vi "Hello.vi"(10 "error in (no error)":errorcluster, 11 "WAMP Client in":refnum<class "WAMP Client.lvclass">) -> (0 "Session ID":u32, 1 "<JSON>":string[](array[string]), 2 "error out":errorcluster, 3 "WAMP Client out":refnum<class "WAMP Client.lvclass">)   [LabVIEW 2020, in "WAMP Client.lvclass"]
uses:
  <userlib>/lvwamp/WAMP Client/WAMP Client.lvclass
  <userlib>/lvwamp/WAMP Client/WAMP Client.lvclass/WAMP Client.ctl
  81aa3083-7749-3644-b591-d0aa62dd8321.vi
  <vilib>/JDP Science/JSONtext/JSON text to Variant.vi
  <vilib>/JDP Science/JSONtext/LVClass Serializer/JSONtext LVClass Serializer.lvclass
  <userlib>/lvwamp/Comm Handlers/ICommHandler/ICommHandler.lvclass
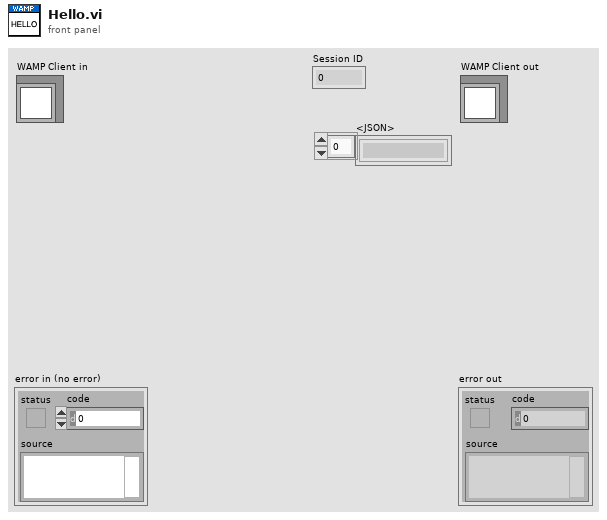
[diagram p1: front panel]
types:
  T1 = typedef "WAMP Client.lvclass/MessageCodes.ctl" = u16
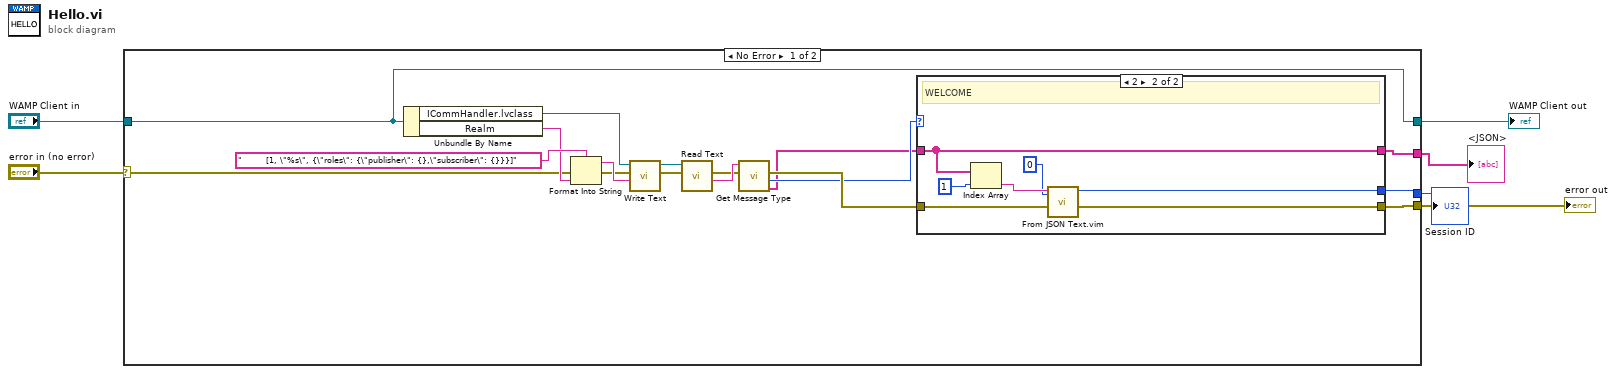
[diagram p0: block diagram]
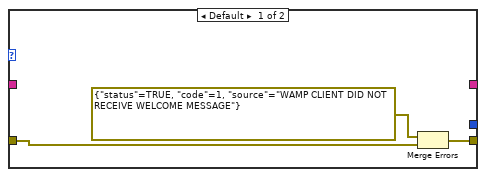
[diagram p2: hidden frame]
diagram:
  n1 = case shown="No Error" "error in (no error)" {
    selector: "error in (no error)" -> [w16 w35]
    tunnel: [w14 w35] -> w5
    tunnel: [w20 w34] -> w3
    tunnel: "WAMP Client in" -> [w20 w34]
    tunnel: [w7 _] -> w2
    tunnel: [w8 _] -> w1
    frame No Error {
      n2 = Unbundle By Name(w20) -> ("ICommHandler.lvclass"=w21:refnum<class "ICommHandler.lvclass">, "Realm"=w18:string)
      n3 = Format Into String(format string="        [1, \"%s\", {\"roles\": {\"publisher\": {},\"subscriber\": {}}}]", error in=w16, w18) -> (resulting string=w17:string, error out=w15:errorcluster)  [unwired: 1 in]
      n4 = call-dynamic "Write Text.vi"("String"=w17, "error in (no error)"=w15, "ICommHandler in"=w21) -> ("error out"=w22:errorcluster, "ICommHandler out"=w23:refnum<class "ICommHandler.lvclass">)  [unwired: 7 in]
      n5 = call-dynamic "Read Text.vi"("error in (no error)"=w22, "ICommHandler in"=w23) -> ("String"=w13:string, "error out"=w12:errorcluster)  [unwired: 5 in, 1 out]
      n6 = call <userlib>:"Get Message Type.vi"("error in (no error)"=w12, "JSON"=w13) -> ("<JSON>"=w9:string[], "Message Codes"=w10:T1, "error out"=w11:errorcluster)  [unwired: 7 in]
      n7 = case shown="2" w10 {
        tunnel: w11 -> [w26 w30]
        tunnel: [w24 w29] -> w14
        tunnel: w9 -> [_ w27]
        tunnel: [_ w28] -> w8
        tunnel: [_ w27] -> w7
        frame Default {
          n8 = Merge Errors(errorcluster {"status"=TRUE, "code"=1, "source"="WAMP CLIENT DID NOT RECEIVE WELCOME MESSAGE"} ("error in"), w26) -> (w24:errorcluster)
        }
        frame 2 {
          # "WELCOME"
          n9 = Index Array(array=w27, index=1) -> (element=w32:string)
          n10 = call "From JSON Text.vim"("Data Type and Default Value"=u32 0, "error in (no error)"=w30, "JSON"=w32) -> ("error out"=w29:errorcluster, "Data out"=w28:u32)  [unwired: 7 in]
        }
      }
    }
    frame Error {
    }
  }
  "error out" <- w5
  "WAMP Client out" <- w3
  "<JSON>" <- w2
  "Session ID" <- w1
